vi "Pulse2GPM.vi"(11 "Pulse/Second":dbl) -> (3 "GPM":dbl)   [LabVIEW 2012]
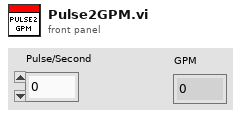
[diagram p1: front panel]
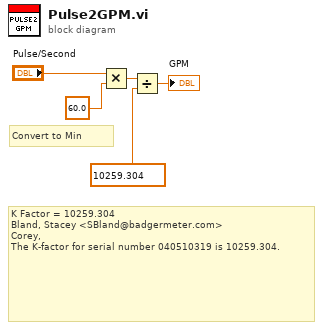
[diagram p0: block diagram]
diagram:
  # "K Factor = 10259.304 \nBland, Stacey <SBland@badgermeter.com> \nCorey,\nThe K-factor for serial number 040510319 is 10259.304."
  # "Convert to Min"
  n1 = Multiply(x="Pulse/Second", y=60.0) -> (x*y=w2:dbl)
  n2 = Divide(x=w2, y=10259.304) -> (x/y=→"GPM":dbl)
